vi "Replace or Add U32.vi"(6 "index (0)":i32, 8 "Element":u32, 11 "Array":u32[](array[numeric])) -> (3 "Array out":u32[](array[numeric]))   [LabVIEW 2020]
doc: "Place U32 element at proper place in Array.\nThis VI is because \"Replace Array Subset\" cannot replace element at position (index) outside of array dimension. I.e. it cannot enlarge array if needed."
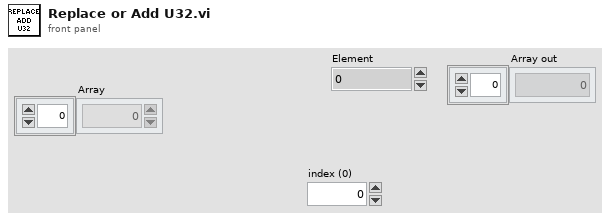
[diagram p1: front panel]
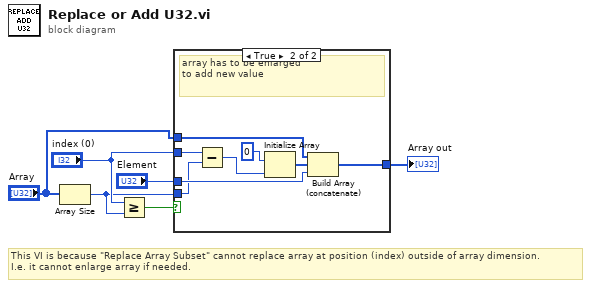
[diagram p0: block diagram]
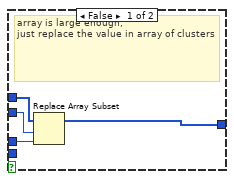
[diagram p2: hidden frame]
diagram:
  # "This VI is because \"Replace Array Subset\" cannot replace array at position (index) outside of array dimension.\nI.e. it cannot enlarge array if needed."
  n1 = Array Size(array="Array") -> (size(s)=w4:i32)
  n2 = Greater Or Equal?(x="index (0)", y=w4) -> (x >= y?=w5:bool)
  n3 = case shown="True" w5 {
    tunnel: "Array" -> [w10 w16]
    tunnel: "index (0)" -> [w9 w14]
    tunnel: "Element" -> [w8 w18]
    tunnel: [w7 w15] -> w1
    tunnel: w4 -> [_ w13]
    frame False {
      # "array is large enough,\njust replace the value in array of clusters"
      n4 = Replace Array Subset(array=w10, new element=w8, index=w9) -> (w7:u32[])
    }
    frame True {
      # "array has to be enlarged\nto add new value"
      n5 = Subtract(x=w14, y=w13) -> (x-y=w12:i32)
      n6 = Initialize Array(u32 0 ("Numeric"), w12) -> (w17:u32[])
      n7 = Build Array (concatenate)(w16, w17, w18) -> (w15:u32[])
    }
  }
  "Array out" <- w1
